vi "SubVI_file_load_index.vi"() -> ()   [LabVIEW 2016]
uses:
  <vilib>/Analysis/baseanly.llb/Mean (DBL).vi
  <vilib>/Waveform/WDTOps.llb/WDT Get Waveform Subset DBL.vi
  <vilib>/Waveform/WDTFileIO.llb/Export Waveforms To Spreadsheet File (1D).vi
  <vilib>/Analysis/NI_AALBase.lvlib
panel:
  out "웨이브폼 그래프":dbl[](graph)
  in  "Stop":bool
  out "error out":errorcluster={"status"=FALSE, "code"=7, "source"=""} caption="에러 출력"
  in  "탭 컨트롤":T1(tab)
  out "Res Acc wf":waveform(dbl)[](graph)
  in  "파일 경로":path=path "C:/TST200/Drop Test Data/ex_raw_data.tdms"
  out "index wf":waveform(dbl)[](graph)=[{"t0"=timestamp(3.62 s since 1904-01-01), "dt"=1e-05, "Y"=array[2000 elements]}, {"t0"=timestamp(3.62 s since 1904-01-01), "dt"=1e-05, "Y"=array[2000 elements]}, {"t0"=timestamp(3.62 s since 1904-01-01), "dt"=1e-05, "Y"=array[2000 elements]}, {"t0"=timestamp(3.62 s since 1904-01-01), "dt"=1e-05, "Y"=array[2000 elements]}, {"t0"=timestamp(3.62 s since 1904-01-01), "dt"=1e-05, "Y"=array[2000 elements]}, {"t0"=timestamp(3.62 s since 1904-01-01), "dt"=1e-05, "Y"=array[2000 elements]}, {"t0"=timestamp(3.62 s since 1904-01-01), "dt"=1e-05, "Y"=array[2000 elements]}, {"t0"=timestamp(3.62 s since 1904-01-01), "dt"=1e-05, "Y"=array[2000 elements]}, {"t0"=timestamp(3.62 s since 1904-01-01), "dt"=1e-05, "Y"=array[2000 elements]}, {"t0"=timestamp(3.62 s since 1904-01-01), "dt"=1e-05, "Y"=array[2000 elements]}, {"t0"=timestamp(3.62 s since 1904-01-01), "dt"=1e-05, "Y"=array[2000 elements]}, {"t0"=timestamp(3.62 s since 1904-01-01), "dt"=1e-05, "Y"=array[2000 elements]}, {"t0"=timestamp(3.62 s since 1904-01-01), "dt"=1e-05, "Y"=array[2000 elements]}, {"t0"=timestamp(3.62 s since 1904-01-01), "dt"=1e-05, "Y"=array[2000 elements]}, {"t0"=timestamp(3.62 s since 1904-01-01), "dt"=1e-05, "Y"=array[2000 elements]}, {"t0"=timestamp(3.62 s since 1904-01-01), "dt"=1e-05, "Y"=array[2000 elements]}]
  in  "index":u32(slide)=181 scale=-1.0..222.0
  out "Acc_peak":dbl=1.6258445790000002 caption="Acc peak"
  out "Acc_time":dbl caption="Acc time" format="%#.1p"
  in  "인덱스":i32
  out "Strain wf":waveform(dbl)[](graph)
  in  "txt save":bool
  out "Strain_ini":dbl[](array[numeric])
  in  "Report":bool
  out "Acc max arrays":dbl[](array[numeric]) format="%#.1f"
  out "Acc peak mean":dbl caption="평균" format="%.1f"
  out "Acc peak max":dbl format="%#.1f"
  out "Acc peak min":dbl format="%#.1f"
  out "cycle number":i32
  out "Res_ini":dbl[](array[numeric])
  out "Strain max 1":dbl format="%#_3e"
  out "Strain max 2":dbl format="%#_3e"
  out "Strain max 3":dbl format="%#_3e"
  out "Strain max 4":dbl format="%#_3e"
  out "Strain min 1":dbl format="%#_3e"
  out "Strain min 2":dbl format="%#_3e"
  out "Strain min 3":dbl format="%#_3e"
  out "Strain min 4":dbl format="%#_3e"
  out "Strain mean 1":dbl format="%#_3e"
  out "Strain mean 2":dbl format="%#_3e"
  out "Strain mean 3":dbl format="%#_3e"
  out "Strain mean 4":dbl format="%#_3e"
  out "Res array":dbl[][](array[numeric]) format="%#.0f"
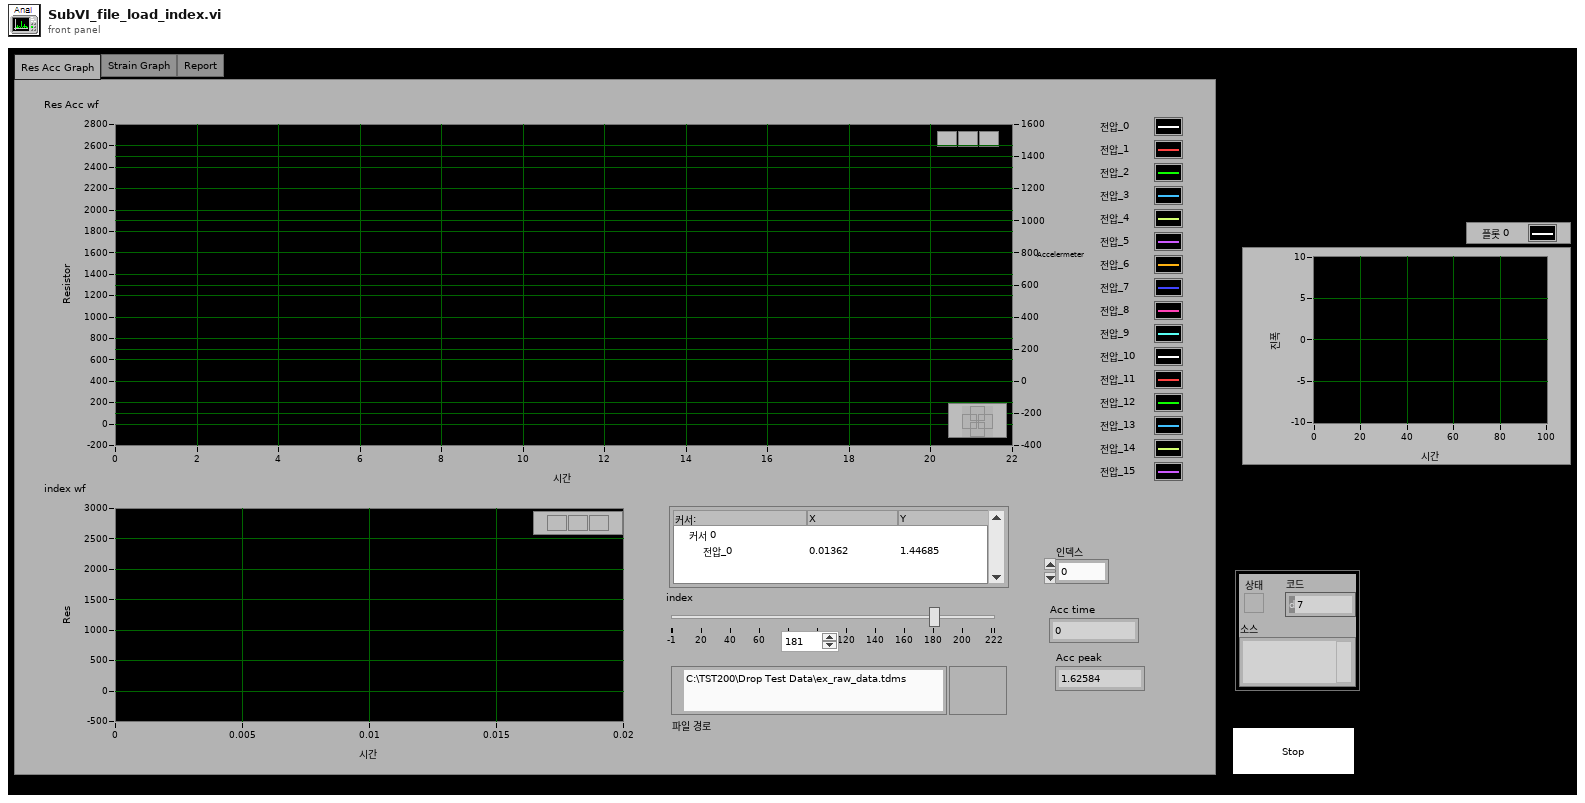
[diagram p1: front panel]
types:
  T1 = enum32{"Res Acc Graph", "Strain Graph", "Report"}
  T2 = enum16{"open", "replace", "create", "open or create", "replace or create", "replace or create with confirmation"}
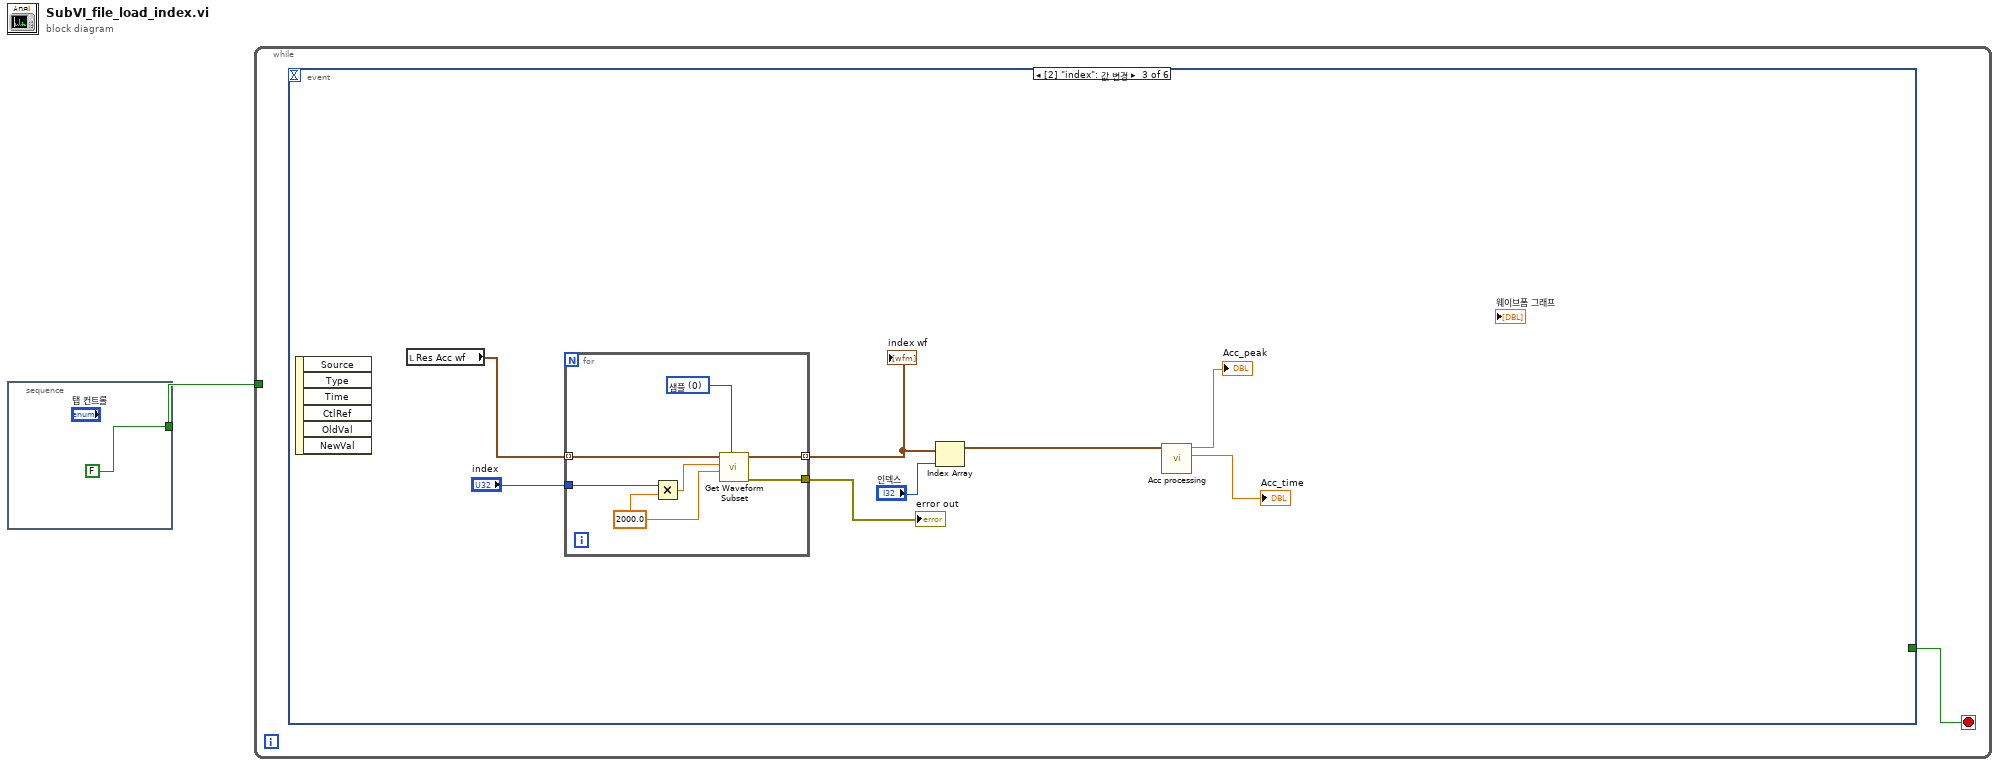
[diagram p0: block diagram]
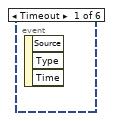
[diagram p2: hidden frame]
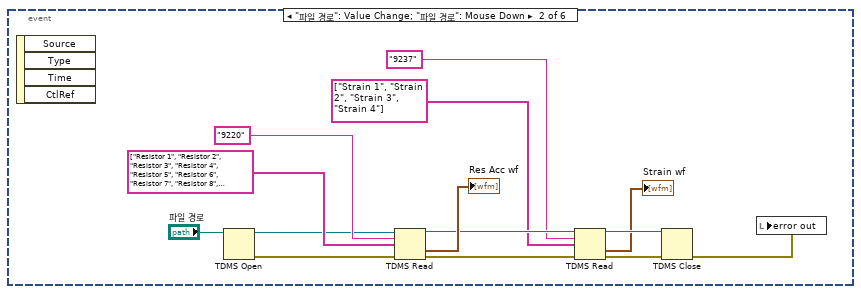
[diagram p3: hidden frame]
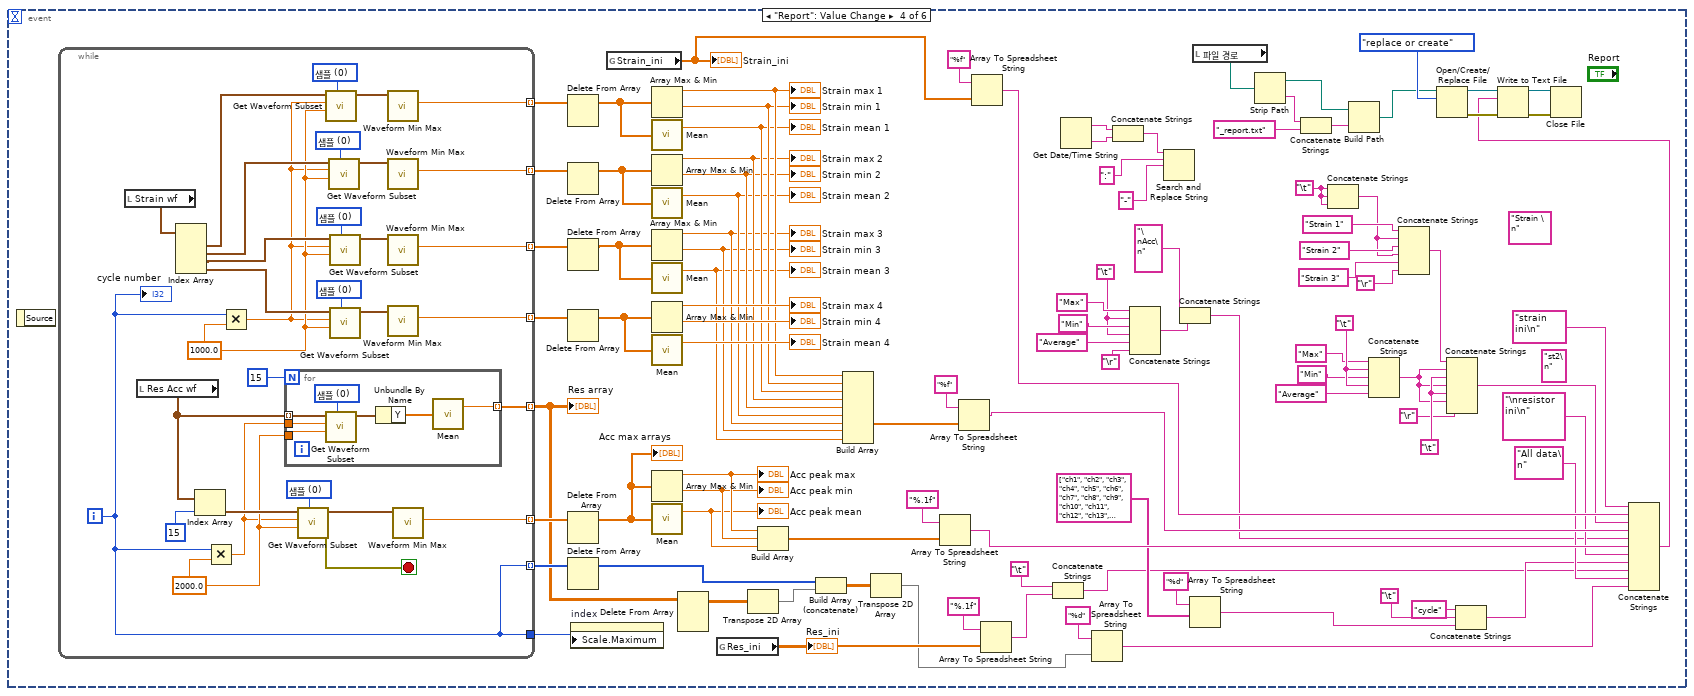
[diagram p4: hidden frame]
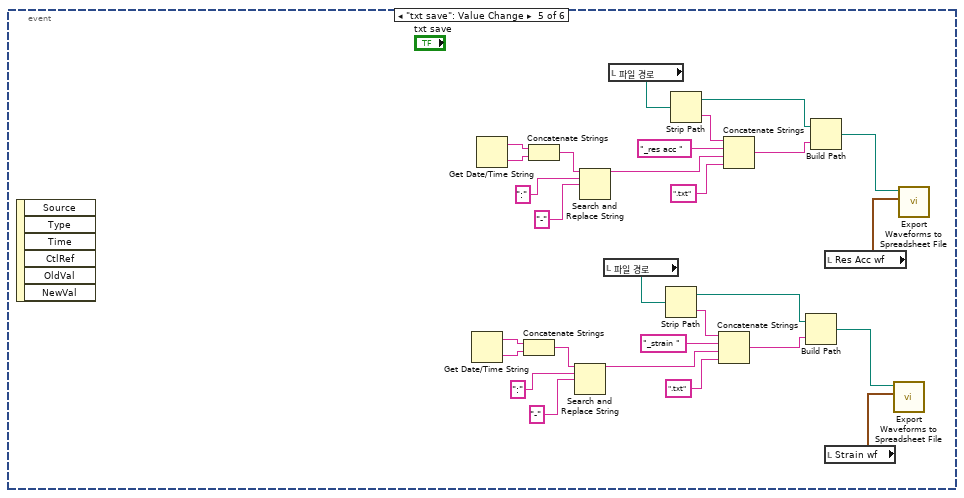
[diagram p5: hidden frame]
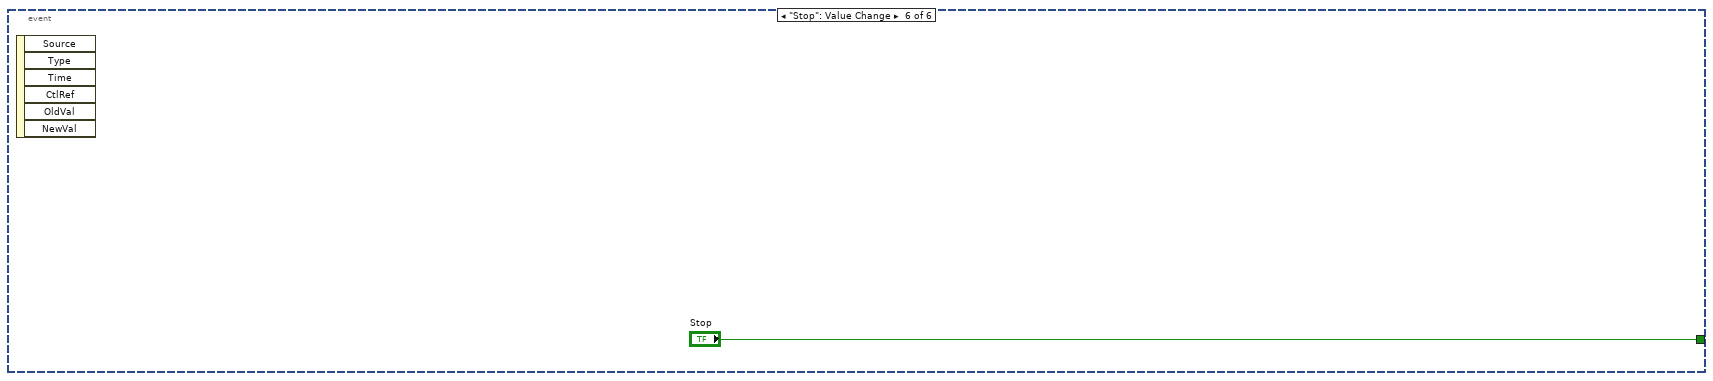
[diagram p6: hidden frame]
diagram:
  n1 = stacked-sequence {
    tunnel: [FALSE ("Deco")] -> w1
    frame #0 {
    }
  }
  n2 = while {
    tunnel: w1 -> [_]
    stop <- w3 stop-if-true
    n3 = event shown="[2] \"index\": 값 변경" {
      selector: _ -> [_ _ _ _ _ _]
      dyn-events: _ -> [_ _ _ _ _ _]
      timeout: _ -> [_ _ _ _ _ _]
      tunnel: [_ _ _ _ _ "Stop"] -> w3
      event Timeout {
        n4 = event-data() -> ()  [unwired: 1 in, 3 out]
      }
      event "파일 경로": Value Change; "파일 경로": Mouse Down {
        n5 = event-data() -> ()  [unwired: 1 in, 4 out]
        n6 = TDMS Open(11:"파일 경로") -> (0:w13:errorcluster, 3:w14:refnum<k34>)  [unwired: 6 in]
        n7 = TDMS Read(0:w14, 5:"9220" ("그룹 이름 입력(제목없음)"), 7:string[] ["Resistor 1", "Resistor 2", "Resistor 3", "Resistor 4", "Resistor 5", "Resistor 6", "Resistor 7", "Resistor 8", "Resistor 9", "Resistor 10", "Resistor 11", "Resistor 12", "Resistor 13", "Resistor 14", "Resistor 15", "Acc"] ("채널 이름 입력(제목없음)"), 11:w13) -> (4:w11:refnum<k34>, 10:→"Res Acc wf":waveform(dbl)[], 15:w9:errorcluster)  [unwired: 4 in, 3 out]
        n8 = TDMS Read(0:w11, 5:"9237" ("그룹 이름 입력(제목없음)"), 7:string[] ["Strain 1", "Strain 2", "Strain 3", "Strain 4"] ("채널 이름 입력(제목없음)"), 11:w9) -> (4:w10:refnum<k34>, 10:→"Strain wf":waveform(dbl)[], 15:w8:errorcluster)  [unwired: 4 in, 3 out]
        n9 = TDMS Close(8:w8, 11:w10) -> (0:w4:errorcluster)  [unwired: 1 out]
        n10 = local write "error out"(w4) -> ()
      }
      event "index": Value Change {
        n11 = event-data() -> ()  [unwired: 1 in, 6 out]
        n12 = local read "Res Acc wf"() -> (w25:waveform(dbl)[])
        n13 = for {
          tunnel: w25 -> [w32] mode=indexing
          tunnel: [w30] -> w22 mode=indexing
          tunnel: "index" -> [w27]
          tunnel: [w26] -> w23
          w29 = 2000.0 ("duration")
          w31 = u16 0 items=["샘플 ", "상대 시간"] ("start/duration format")
          n14 = Multiply(x=w27, y=w29) -> (x*y=w28:dbl)
          n15 = call-poly <vilib>:"Get Waveform Subset.vi"("start/duration format"=w31, "duration"=w29, "start samples/time"=w28, "waveform in"=w32) -> ("error out"=w26:errorcluster, "waveform out"=w30:waveform(dbl))  [unwired: 2 in, 2 out]
        }
        "index wf" <- w22
        "error out" <- w23
        n16 = Index Array(array=w22, index="인덱스") -> (element=w20:waveform(dbl))
        n17 = call "Acc processing.vi"("Raw_acc"=w20) -> ("Acc_time"=→"Acc_time":dbl, "Acc_peak"=→"Acc_peak":dbl)  [unwired: 9 in]
      }
      event "Report": Value Change {
        w38 = "\t"
        w59 = "\t"
        w62 = "\t"
        (unwired) "Strain \n" ("문자열")
        w69 = "\t"
        (unwired) "st2\n" ("문자열")
        n18 = event-data() -> ()  [unwired: 1 in, 1 out]
        n19 = while {
          tunnel: [w159] -> w130 mode=indexing
          tunnel: [w131] -> w128
          tunnel: [w154] -> w127 mode=indexing
          tunnel: [w153] -> w126 mode=indexing
          tunnel: [w152] -> w125 mode=indexing
          tunnel: [w151] -> w124 mode=indexing
          tunnel: [w132] -> w49 mode=indexing
          tunnel: [w131] -> w51 mode=indexing
          i -> [w131]
          stop <- w137 stop-if-true
          w148 = u16 0 items=["샘플 ", "상대 시간"] ("start/duration format")
          w149 = u16 0 items=["샘플 ", "상대 시간"] ("start/duration format")
          w150 = u16 0 items=["샘플 ", "상대 시간"] ("start/duration format")
          w143 = 1000.0 ("duration")
          w155 = u16 0 items=["샘플 ", "상대 시간"] ("start/duration format")
          w134 = 2000.0 ("duration")
          w161 = u16 0 items=["샘플 ", "상대 시간"] ("start/duration format")
          n20 = local read "Strain wf"() -> (w156:waveform(dbl)[])
          n21 = local read "Res Acc wf"() -> (w136:waveform(dbl)[])
          n22 = Index Array(array=w156) -> (element #1=w144:waveform(dbl), element #2=w145:waveform(dbl), element #3=w146:waveform(dbl), element #4=w147:waveform(dbl))  [unwired: 4 in]
          n23 = Index Array(array=w136, index=15 ("인덱스")) -> (element=w157:waveform(dbl))
          n24 = Multiply(x=w131, y=w134) -> (x*y=w133:dbl)
          n25 = Multiply(x=w131, y=w143) -> (x*y=w142:dbl)
          n26 = for {
            N: 15 -> [_]
            tunnel: w136 -> [w165] mode=indexing
            tunnel: w134 -> [w167]
            tunnel: w133 -> [w166]
            tunnel: [w162] -> w132 mode=indexing
            w168 = u16 0 items=["샘플 ", "상대 시간"] ("start/duration format")
            n27 = call-poly <vilib>:"Get Waveform Subset.vi"("start/duration format"=w168, "duration"=w167, "start samples/time"=w166, "waveform in"=w165) -> ("waveform out"=w164:waveform(dbl))  [unwired: 2 in, 3 out]
            n28 = Unbundle By Name(w164) -> ("Y"=w163:dbl[])
            n29 = call-poly <vilib>:"Mean.vi"("X"=w163) -> ("mean"=w162:dbl)  [unwired: 1 out]
          }
          n30 = call-poly <vilib>:"Get Waveform Subset.vi"("start/duration format"=w161, "duration"=w134, "start samples/time"=w133, "waveform in"=w157) -> ("error out"=w137:errorcluster, "waveform out"=w160:waveform(dbl))  [unwired: 2 in, 2 out]
          n31 = call-poly <vilib>:"Get Waveform Subset.vi"("start/duration format"=w148, "duration"=w143, "start samples/time"=w142, "waveform in"=w144) -> ("waveform out"=w141:waveform(dbl))  [unwired: 2 in, 3 out]
          n32 = call-poly <vilib>:"Get Waveform Subset.vi"("start/duration format"=w149, "duration"=w143, "start samples/time"=w142, "waveform in"=w145) -> ("waveform out"=w140:waveform(dbl))  [unwired: 2 in, 3 out]
          n33 = call-poly <vilib>:"Get Waveform Subset.vi"("start/duration format"=w150, "duration"=w143, "start samples/time"=w142, "waveform in"=w146) -> ("waveform out"=w139:waveform(dbl))  [unwired: 2 in, 3 out]
          n34 = call-poly <vilib>:"Get Waveform Subset.vi"("start/duration format"=w155, "duration"=w143, "start samples/time"=w142, "waveform in"=w147) -> ("waveform out"=w138:waveform(dbl))  [unwired: 2 in, 3 out]
          n35 = call <vilib>:"Waveform Min Max.vi"("waveform in"=w141) -> ("Y max"=w151:dbl)  [unwired: 5 in, 5 out]
          n36 = call <vilib>:"Waveform Min Max.vi"("waveform in"=w140) -> ("Y max"=w152:dbl)  [unwired: 5 in, 5 out]
          n37 = call <vilib>:"Waveform Min Max.vi"("waveform in"=w139) -> ("Y max"=w153:dbl)  [unwired: 5 in, 5 out]
          n38 = call <vilib>:"Waveform Min Max.vi"("waveform in"=w138) -> ("Y max"=w154:dbl)  [unwired: 5 in, 5 out]
          n39 = call <vilib>:"Waveform Min Max.vi"("waveform in"=w160) -> ("Y max"=w159:dbl)  [unwired: 5 in, 5 out]
          "cycle number" <- w131
        }
        "Res array" <- w49
        n40 = Delete From Array(array=w124) -> (array with subset deleted=w120:dbl[])  [unwired: 2 in, 1 out]
        n41 = Delete From Array(array=w125) -> (array with subset deleted=w121:dbl[])  [unwired: 2 in, 1 out]
        n42 = Delete From Array(array=w126) -> (array with subset deleted=w122:dbl[])  [unwired: 2 in, 1 out]
        n43 = Delete From Array(array=w127) -> (array with subset deleted=w123:dbl[])  [unwired: 2 in, 1 out]
        n44 = Delete From Array(array=w130) -> (array with subset deleted=w129:dbl[])  [unwired: 2 in, 1 out]
        "Acc max arrays" <- w129
        n45 = Delete From Array(array=w51) -> (array with subset deleted=w50:i32[])  [unwired: 2 in, 1 out]
        n46 = property on="index" class="Slide (엄격한)"("Scale.Maximum"=w128) -> ()  [unwired: 2 in, 2 out]
        n47 = global read "글로벌_Config Parameter.vi" "Strain_ini"() -> (w92:dbl[])
        "Strain_ini" <- w92
        n48 = Array Max & Min(array=w120) -> (max value=w116:dbl, min value=w115:dbl)  [unwired: 2 out]
        "Strain max 1" <- w116
        "Strain min 1" <- w115
        n49 = call-poly <vilib>:"Mean.vi"("X"=w120) -> ("mean"=w114:dbl)  [unwired: 1 out]
        "Strain mean 1" <- w114
        n50 = Array Max & Min(array=w121) -> (max value=w113:dbl, min value=w112:dbl)  [unwired: 2 out]
        "Strain max 2" <- w113
        "Strain min 2" <- w112
        n51 = call-poly <vilib>:"Mean.vi"("X"=w121) -> ("mean"=w111:dbl)  [unwired: 1 out]
        "Strain mean 2" <- w111
        n52 = Array Max & Min(array=w122) -> (max value=w110:dbl, min value=w109:dbl)  [unwired: 2 out]
        "Strain max 3" <- w110
        "Strain min 3" <- w109
        n53 = call-poly <vilib>:"Mean.vi"("X"=w122) -> ("mean"=w108:dbl)  [unwired: 1 out]
        "Strain mean 3" <- w108
        n54 = Array Max & Min(array=w123) -> (max value=→"Strain max 4":dbl, min value=→"Strain min 4":dbl)  [unwired: 2 out]
        n55 = call-poly <vilib>:"Mean.vi"("X"=w123) -> ("mean"=→"Strain mean 4":dbl)  [unwired: 1 out]
        n56 = Array Max & Min(array=w129) -> (max value=w107:dbl, min value=w106:dbl)  [unwired: 2 out]
        "Acc peak max" <- w107
        "Acc peak min" <- w106
        n57 = call-poly <vilib>:"Mean.vi"("X"=w129) -> ("mean"=w105:dbl)  [unwired: 1 out]
        "Acc peak mean" <- w105
        n58 = Delete From Array(array=w49) -> (array with subset deleted=w48:dbl[][])  [unwired: 3 in, 1 out]
        n59 = global read "글로벌_Config Parameter.vi" "Res_ini"() -> (w94:dbl[])
        "Res_ini" <- w94
        n60 = Transpose 2D Array(2D array=w48) -> (transposed array=w81:dbl[][])
        n61 = Build Array(w107, w106, w105) -> (w98:dbl[])
        n62 = Build Array (concatenate)(w50, w81) -> (w82:dbl[][])
        n63 = Build Array(w116, w115, w114, w113, w112, w111, w110, w109, w108) -> (w96:dbl[])
        n64 = Transpose 2D Array(2D array=w82) -> (transposed array=w80:dbl[][])
        n65 = Array To Spreadsheet String(array=w98, 3:"%.1f" ("포맷 문자열")) -> (spreadsheet string=w88:string)  [unwired: 1 in]
        n66 = Array To Spreadsheet String(array=w96, 3:"%f" ("포맷 문자열")) -> (spreadsheet string=w89:string)  [unwired: 1 in]
        n67 = Array To Spreadsheet String(array=w92, 3:"%f" ("포맷 문자열")) -> (spreadsheet string=w91:string)  [unwired: 1 in]
        n68 = Array To Spreadsheet String(array=w94, 3:"%.1f" ("포맷 문자열")) -> (spreadsheet string=w47:string)  [unwired: 1 in]
        n69 = Concatenate Strings("\t", w47) -> (w46:string)
        n70 = Get Date/Time String() -> (date string=w35:string, time string=w34:string)  [unwired: 3 in]
        n71 = Array To Spreadsheet String(array=w80, 3:"%d" ("포맷 문자열")) -> (spreadsheet string=w84:string)  [unwired: 1 in]
        n72 = Concatenate Strings(w35, w34) -> (w36:string)
        n73 = Concatenate Strings("Max" ("문자열"), w69, "Min" ("문자열"), w69, "Average" ("문자열"), "\r") -> (w66:string)
        n74 = Search and Replace String(input string=w36, search string=":" ("검색 문자열"), replace string="-" ("대체 문자열(\"\")")) -> ()  [unwired: 5 in, 4 out]
        n75 = Concatenate Strings("\nAcc\n" ("문자열"), w66) -> (w64:string)
        n76 = Array To Spreadsheet String(array=string[] ["ch1", "ch2", "ch3", "ch4", "ch5", "ch6", "ch7", "ch8", "ch9", "ch10", "ch11", "ch12", "ch13", "ch14", "ch15"], 3:"%d" ("포맷 문자열")) -> (spreadsheet string=w53:string)  [unwired: 1 in]
        n77 = local read "파일 경로"() -> (w77:path)
        n78 = Strip Path(path=w77) -> (stripped path=w76:path, name=w75:string)
        n79 = Concatenate Strings(w75, "_report.txt" ("문자열")) -> (w73:string)
        n80 = Concatenate Strings(w38, w38, w38) -> (w41:string)
        n81 = Build Path(base path=w76, name or relative path=w73) -> (appended path=w72:path)
        n82 = Concatenate Strings("Max" ("문자열"), w62, "Min" ("문자열"), w62, "Average" ("문자열")) -> (w58:string)
        n83 = Concatenate Strings("Strain 1" ("문자열"), w41, "Strain 2" ("문자열"), w41, "Strain 3" ("문자열"), "\r") -> (w39:string)
        n84 = Open/Create/Replace File(file path (use dialog)=w72, operation (0:open)=T2."replace or create" ("동작(0:open)")) -> (refnum out=w101:refnum<file>, error out=w103:errorcluster)  [unwired: 4 in, 1 out]
        n85 = Concatenate Strings(w39, w58, w59, w58, w59, w58, "\r") -> (w56:string)
        n86 = Concatenate Strings("cycle" ("문자열"), "\t", w53) -> (w52:string)
        n87 = Concatenate Strings("strain ini\n" ("문자열"), w91, w56, w89, w64, w88, "\nresistor ini\n" ("문자열"), w52, w46, "All data\n" ("문자열"), w84) -> (w83:string)
        n88 = Write to Text File(file (use dialog)=w101, text=w83, error in=w103) -> (refnum out=w100:refnum<file>, error out=w102:errorcluster)  [unwired: 1 in, 1 out]
        n89 = Close File(refnum=w100, error in=w102) -> ()  [unwired: 2 out]
      }
      event "txt save": Value Change {
        n90 = event-data() -> ()  [unwired: 1 in, 6 out]
        n91 = Get Date/Time String() -> (date string=w175:string, time string=w174:string)  [unwired: 3 in]
        n92 = Get Date/Time String() -> (date string=w190:string, time string=w191:string)  [unwired: 3 in]
        n93 = Concatenate Strings(w175, w174) -> (w176:string)
        n94 = Concatenate Strings(w190, w191) -> (w189:string)
        n95 = Search and Replace String(input string=w176, search string=":" ("검색 문자열"), replace string="-" ("대체 문자열(\"\")")) -> (result string=w172:string)  [unwired: 5 in, 3 out]
        n96 = Search and Replace String(input string=w189, search string=":" ("검색 문자열"), replace string="-" ("대체 문자열(\"\")")) -> (result string=w193:string)  [unwired: 5 in, 3 out]
        n97 = local read "파일 경로"() -> (w180:path)
        n98 = local read "파일 경로"() -> (w185:path)
        n99 = Strip Path(path=w180) -> (stripped path=w170:path, name=w179:string)
        n100 = Strip Path(path=w185) -> (stripped path=w195:path, name=w186:string)
        n101 = Concatenate Strings(w179, "_strain " ("문자열"), w172, ".txt" ("문자열")) -> (w169:string)
        n102 = Concatenate Strings(w186, "_res acc " ("문자열"), w193, ".txt" ("문자열")) -> (w196:string)
        n103 = Build Path(base path=w170, name or relative path=w169) -> (appended path=w181:path)
        n104 = Build Path(base path=w195, name or relative path=w196) -> (appended path=w184:path)
        n105 = local read "Res Acc wf"() -> (w183:waveform(dbl)[])
        n106 = local read "Strain wf"() -> (w182:waveform(dbl)[])
        n107 = call-poly <vilib>:"Export Waveforms to Spreadsheet File.vi"("waveforms"=w182, "file path (dialog if empty)"=w181) -> ()  [unwired: 8 in, 2 out]
        n108 = call-poly <vilib>:"Export Waveforms to Spreadsheet File.vi"("waveforms"=w183, "file path (dialog if empty)"=w184) -> ()  [unwired: 8 in, 2 out]
      }
      event "Stop": Value Change {
        n109 = event-data() -> ()  [unwired: 1 in, 6 out]
      }
    }
  }
